vi "fgv_gridmap_process-val.vi"(7 "cmd":T3, 11 "p-val":T2) -> (3 "p-val  2":T2)   [LabVIEW 2019]
uses:
  Ctrl/cmd_common.ctl
  <vilib>/Analysis/Matrix/Datatypes/RealMatrix.ctl
  <vilib>/Analysis/Matrix/NI_Matrix.lvlib
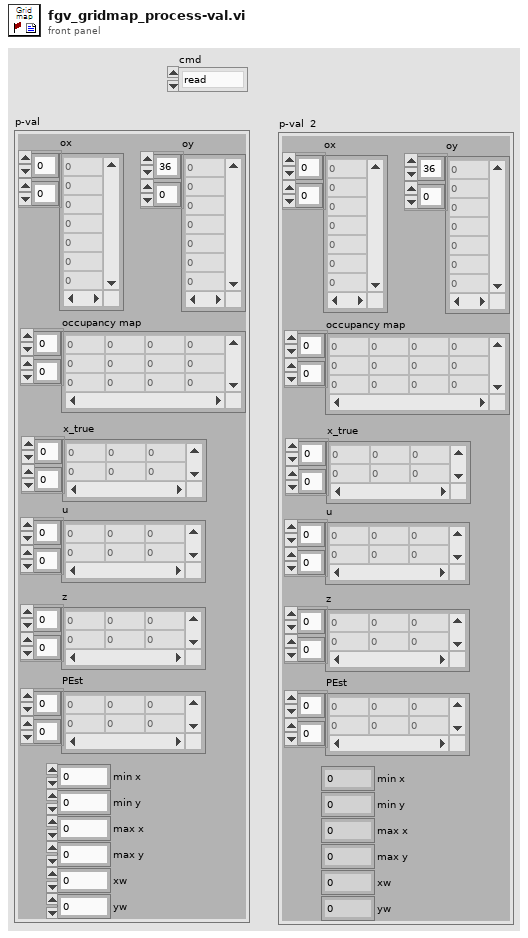
[diagram p1: front panel]
types:
  T1 = typedef "NI_Matrix.lvlib/RealMatrix.ctl" = dbl[][]
  T2 = cluster{"ox":T1, "oy":T1, "occupancy map":T1, "x_true":T1, "u":T1, "z":T1, "PEst":T1, "min x":dbl, "min y":dbl, "max x":dbl, "max y":dbl, "yw":i32, "xw":i32}
  T3 = typedef "cmd_common.ctl" = enum16{"read", "write"}
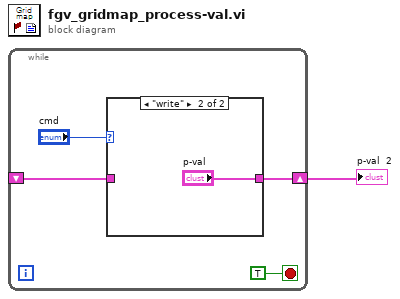
[diagram p0: block diagram]
diagram:
  n1 = while {
    shift-right: [w3] -> w1
    shift-left: _ -> [w2]
    stop <- TRUE stop-if-true
    n2 = case shown="\"write\"" "cmd" {
      tunnel: [w6 "p-val"] -> w3
      tunnel: w2 -> [w6 _]
      frame "read", Default {
      }
      frame "write" {
      }
    }
  }
  "p-val  2" <- w1
